vi "Curtin1_ErrorDialog.vi"(8 "error in (no error)":errorcluster, 11 "String":string) -> (2 "true":bool)   [LabVIEW 2022 SP3]
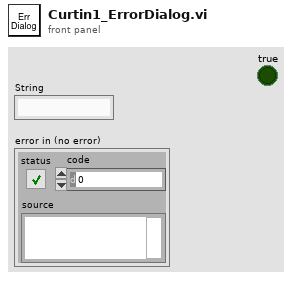
[diagram p1: front panel]
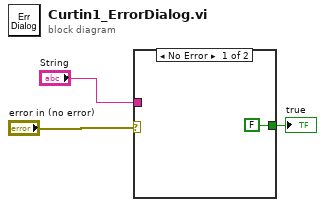
[diagram p0: block diagram]
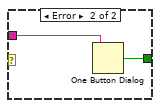
[diagram p2: hidden frame]
diagram:
  n1 = case shown="No Error" "error in (no error)" {
    tunnel: "String" -> [_ w6]
    tunnel: [FALSE ("true") w5] -> w1
    frame No Error {
    }
    frame Error {
      n2 = One Button Dialog(message=w6) -> (true=w5:bool)  [unwired: 1 in]
    }
  }
  "true" <- w1
